vi "Remove_FF_lone_spikes.vi"(3 "ADC Frequency Hz":dbl=1000.0 format="%.2f", 4 "Bkgnd variance":dbl format="%.6f", 5 "AIC index":i32, 6 "Time Trace":dbl[](array[numeric])) -> (0 "No Removed":i32, 2 "Filtered Time Trace":dbl[](array[numeric]))   [LabVIEW 2013]
uses:
  Globals/Meas_global.vi
panel:
  out "Time Trace":dbl[][](graph)
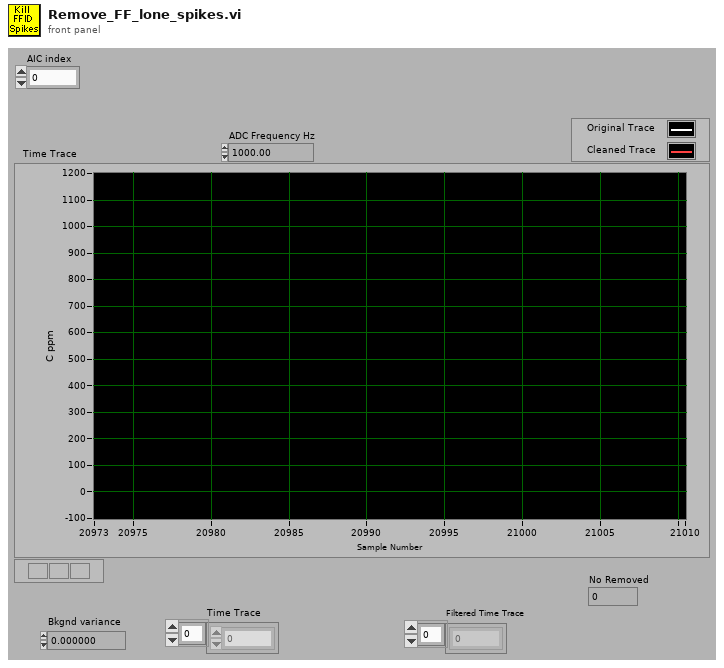
[diagram p1: front panel]
types:
  T1 = typedef "Analysis_info_cluster.ctl" = cluster{"Colour":u32, "Inst type":T2, "Inst name":string, "Symbol":string, "Code name":string, "Extra Info":string, "Inst Array":T3, "Extra Titles":string[], "Extra Values":string[], "U":dbl, "u^2":dbl, "u^3":dbl, "u^4":dbl, "Skew_u":dbl, "Kurt_u":dbl, "Sd Error in Mean":dbl, "% u'/U":dbl, "X":dbl, "Y":dbl, "Z":dbl, "Timescale integral to 25%":dbl, "Sd Error in Variance":dbl, "Calib File":path, "Calib Constants":dbl[], "Output Position":bool, "Full Stats":bool, "Av Sampling Rate":dbl, "Av No of Samples":dbl, "Total Meas Time (s)":dbl, "ADAM Ch Name":string}
  T2 = typedef "Inst_type.ctl" = enum16{"Propeller anemometer", "Raw voltage", "Pressure Transducer", "Pitot-static tube", "Preston tube", "Hot wire", "Cross wire 1", "Cross wire 2", "Generic Linear", "Generic Polynomial", "Generic BackPoly", "Fast FID", "Thermocouple", "Cold wire", "Pulsed Wire", "LDA Vel", "LDA Tran time", "LDA Arr time"}
  T3 = typedef "Instrument_Array.ctl" = enum16{"PWA", "LDA", "Analogue"}
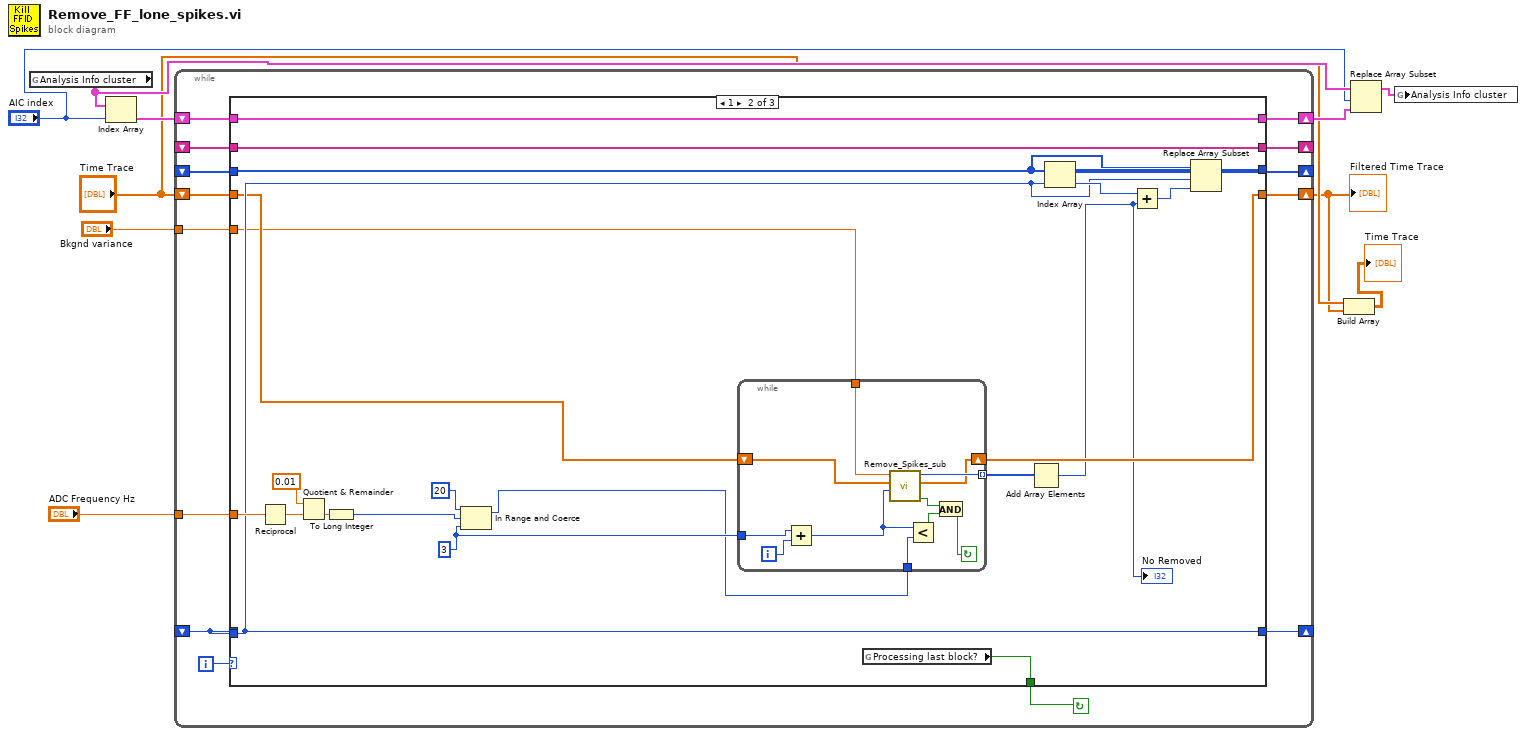
[diagram p0: block diagram]
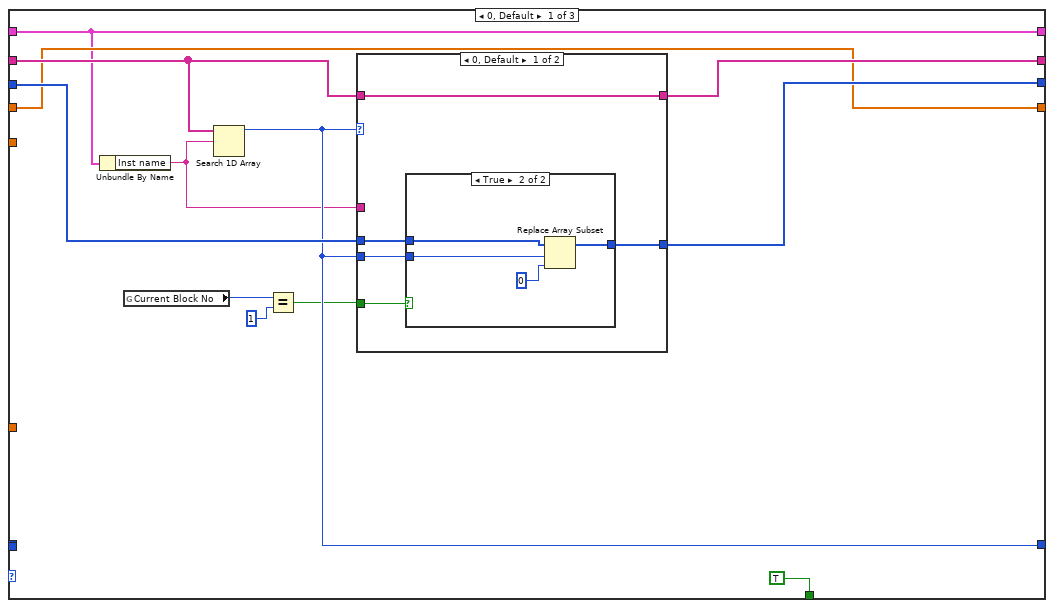
[diagram p2: hidden frame]
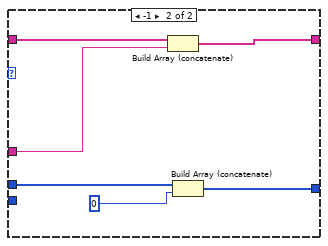
[diagram p4: hidden frame]
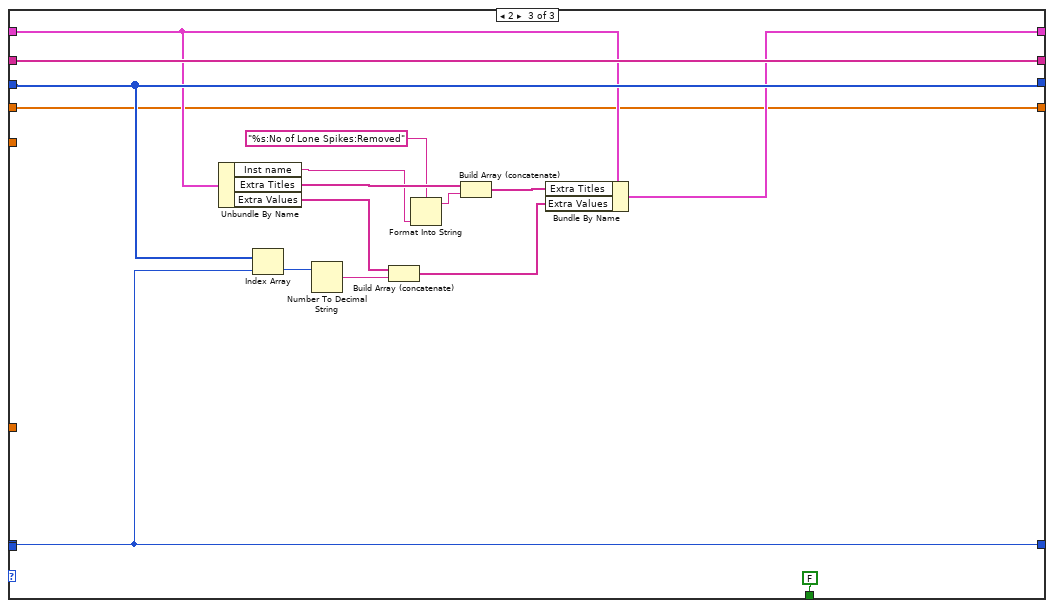
[diagram p5: hidden frame]
diagram:
  n1 = global read "Meas_global.vi" "Analysis Info cluster"() -> (w7:T1[])
  n2 = Index Array(array=w7, index="AIC index") -> (element=w8:T1)
  n3 = while {
    shift-left: _ -> [w21]
    shift-right: [w23] -> _
    shift-right: [w19] -> _
    shift-left: _ -> [w20]
    shift-right: [w17] -> _
    shift-left: _ -> [w18]
    shift-right: [w15] -> w6
    shift-left: w8 -> [w16]
    tunnel: "Bkgnd variance" -> [w14]
    shift-right: [w12] -> w2
    shift-left: "Time Trace" -> [w13]
    tunnel: "ADC Frequency Hz" -> [w11]
    i -> [w24]
    stop <- w22 continue-if-true
    n4 = case shown="1" w24 {
      tunnel: [w29 w63 w98] -> w23
      tunnel: [TRUE w62 FALSE ("Processing last block?")] -> w22
      tunnel: w21 -> [_ _ w98]
      tunnel: w21 -> [_ w63 _]
      tunnel: w20 -> [w33 w73 w96]
      tunnel: [w32 w73 w96] -> w19
      tunnel: w18 -> [w31 w72 w95]
      tunnel: [w30 w70 w95] -> w17
      tunnel: w16 -> [w26 w69 w92]
      tunnel: [w26 w69 w94] -> w15
      tunnel: w14 -> [_ w53 _]
      tunnel: w13 -> [w27 w59 w88]
      tunnel: [w27 w58 w88] -> w12
      tunnel: w11 -> [_ w67 _]
      frame 0, Default {
        n5 = Unbundle By Name(w26) -> ("Inst name"=w25:string)
        n6 = global read "Meas_global.vi" "Current Block No"() -> (w35:i32)
        n7 = Search 1D Array(1D array=w33, element=w25) -> (index of element=w29:i32)  [unwired: 1 out]
        n8 = Equal?(x=w35, y=1) -> (x = y?=w28:bool)
        n9 = case shown="0, Default" w29 {
          tunnel: w33 -> [w41 w52]
          tunnel: w25 -> [_ w51]
          tunnel: [w41 w50] -> w32
          tunnel: w31 -> [w40 w49]
          tunnel: [w39 w48] -> w30
          tunnel: w29 -> [w38 _]
          tunnel: w28 -> [w37 _]
          frame 0, Default {
            n10 = case shown="True" w37 {
              tunnel: w40 -> [w42 w46]
              tunnel: [w42 w45] -> w39
              tunnel: w38 -> [_ w44]
              frame False {
              }
              frame True {
                n11 = Replace Array Subset(array=w46, new element=0, index=w44) -> (w45:i32[])
              }
            }
          }
          frame -1 {
            n12 = Build Array (concatenate)(w52, w51) -> (w50:string[])
            n13 = Build Array (concatenate)(w49, 0) -> (w48:i32[])
          }
        }
      }
      frame 1 {
        w55 = 3 ("lower limit")
        n14 = Reciprocal(x=w67) -> (1/x=w65:dbl)
        n15 = Quotient & Remainder(x=0.01, y=w65) -> (floor(x/y)=w64:dbl)  [unwired: 1 out]
        n16 = To Long Integer(number=w64) -> (32bit integer=w60:i32)
        n17 = In Range and Coerce(upper limit=20, x=w60, lower limit=w55) -> (coerced(x)=w54:i32)  [unwired: 1 out]
        n18 = while {
          tunnel: [w84] -> w57 mode=indexing
          shift-right: [w83] -> w58
          shift-left: w59 -> [w78]
          tunnel: w55 -> [w81]
          tunnel: w54 -> [w79]
          tunnel: w53 -> [w74]
          i -> [w82]
          stop <- w75 continue-if-true
          n19 = Add(x=w81, y=w82) -> (x+y=w80:i32)
          n20 = call "Remove_Spikes_sub.vi"("Number of samples"=w80, "Time Trace in"=w78, "Bkgnd Variance"=w74) -> ("Checked"=w77:bool, "Time Trace out"=w83:dbl[], "Numeric out"=w84:i32)  [unwired: 6 in]
          n21 = Less?(x=w80, y=w79) -> (x < y?=w76:bool)
          n22 = And(x=w77, y=w76) -> (x .and. y?=w75:bool)
        }
        n23 = global read "Meas_global.vi" "Processing last block?"() -> (w62:bool)
        n24 = Add Array Elements(numeric array=w57) -> (sum=w56:i32)
        "No Removed" <- w56
        n25 = Index Array(array=w72, index=w63) -> (element=w71:i32)
        n26 = Add(x=w71, y=w56) -> (x+y=w68:i32)
        n27 = Replace Array Subset(array=w72, new element=w68, index=w63) -> (w70:i32[])
      }
      frame 2 {
        n28 = Unbundle By Name(w92) -> ("Inst name"=w86:string, "Extra Titles"=w91:string[], "Extra Values"=w90:string[])
        n29 = Index Array(array=w95, index=w98) -> (element=w97:i32)
        n30 = Number To Decimal String(number=w97) -> (decimal integer string=w99:string)  [unwired: 1 out]
        n31 = Build Array (concatenate)(w90, w99) -> (w89:string[])
        n32 = Format Into String(format string="%s:No of Lone Spikes:Removed", w86) -> (resulting string=w87:string)  [unwired: 2 in, 1 out]
        n33 = Build Array (concatenate)(w91, w87) -> (w93:string[])
        n34 = Bundle By Name(cluster=w92, "Extra Titles"=w93, "Extra Values"=w89) -> (w94:T1)
      }
    }
  }
  "Filtered Time Trace" <- w2
  n35 = Build Array("Time Trace", w2) -> (→"Time Trace":dbl[][])
  n36 = Replace Array Subset(array=w7, new element=w6, index="AIC index") -> (w4:T1[])
  n37 = global write "Meas_global.vi" "Analysis Info cluster"(w4) -> ()
